vi "To String.vi"(8 "error in (no error)":errorcluster, 11 "Double Float in":refnum<class "Abs_Time.lvclass">) -> (0 "error out":errorcluster, 2 "String":string, 3 "Double Float out":refnum<class "Abs_Time.lvclass">)   [LabVIEW 2021, in "Abs_Time.lvclass"]
uses:
  Abs_Time.lvclass
  C:/TSA/LV_Abstract/Source/Abs_Types/Numeric/Abs_Numeric.lvclass
  Numeric/Abs_Numeric.lvclass/Abs_Numeric.ctl
  Abs_Time.lvclass/Abs_Time.ctl
  Numeric/Properties/Read Units.vi
  Properties/Read UTC Time For String Format.vi
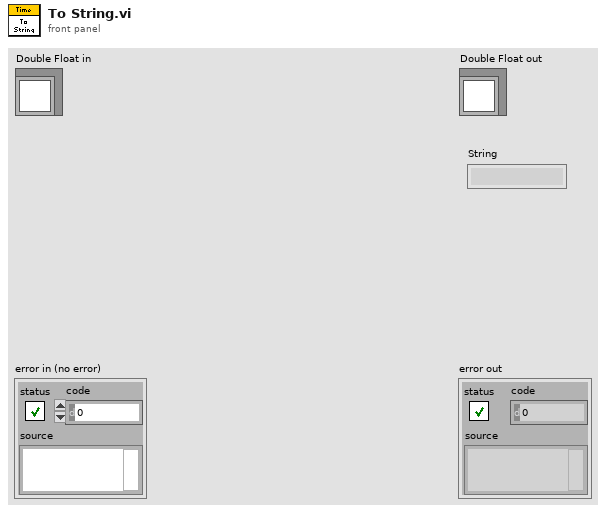
[diagram p1: front panel]
types:
  T1 = typedef "Abs_Time.lvclass/Type.ctl" = timestamp
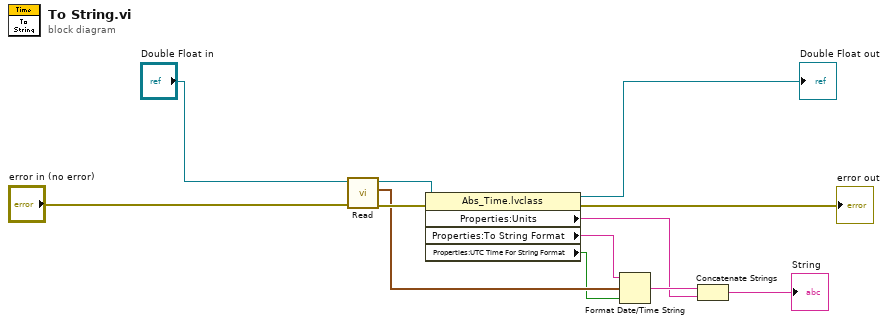
[diagram p0: block diagram]
diagram:
  n1 = call-dynamic "Read.vi"("error in (no error)"="error in (no error)", "Double Float.lvclass_340760 in"="Double Float in") -> ("error out"=w5:errorcluster, "Value"=w4:T1, "Double Float.lvclass_340760 out"=w6:refnum<class "Abs_Time.lvclass">)  [unwired: 7 in]
  n2 = property class="Abs_Time.lvclass"(reference=w6, error in=w5) -> (reference out=→"Double Float out":refnum<class "Abs_Time.lvclass">, error out=→"error out":errorcluster, "Properties:Units"=w1:string, "Properties:To String Format"=w3:string, "Properties:UTC Time For String Format"=w2:bool)
  n3 = Format Date/Time String(time format string (%c)=w3, seconds (now)=w4, UTC format=w2) -> (date/time string=w7:string)
  n4 = Concatenate Strings(w7, w1) -> (→"String":string)
